vi "enable_channel.vi"(4 "Delay":i32, 6 "V clip":i32, 7 "V att":i32=4095, 8 "error in":errorcluster, 9 "Channel":i32(ring) items=["sendCommand"=9, "FPGA_writeRegister"=3, "FPGA_readRegister"=2, "uC_writeRegister"=1, "uC_readRegister"=0], 10 "id_in":i32, 11 "connection ID":refnum<k5>) -> (0 "error out":errorcluster, 1 "id_out":i32, 3 "connection ID out":refnum<k5>)   [LabVIEW 2009]
doc: "This VI sends a command to the Integration Board and provides the received data when necessary."
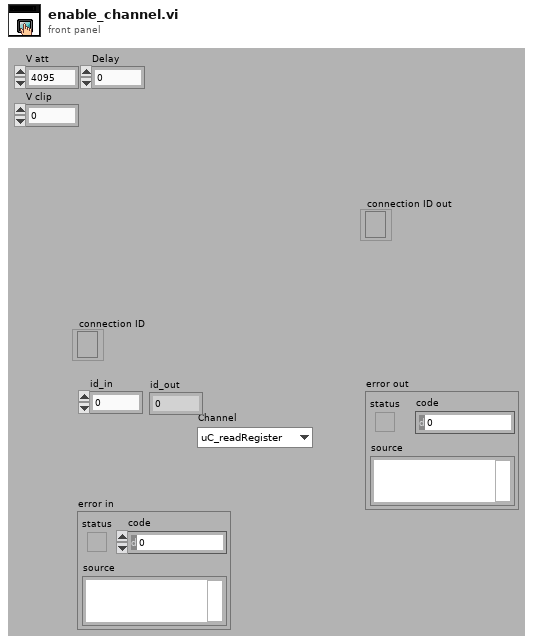
[diagram p1: front panel]
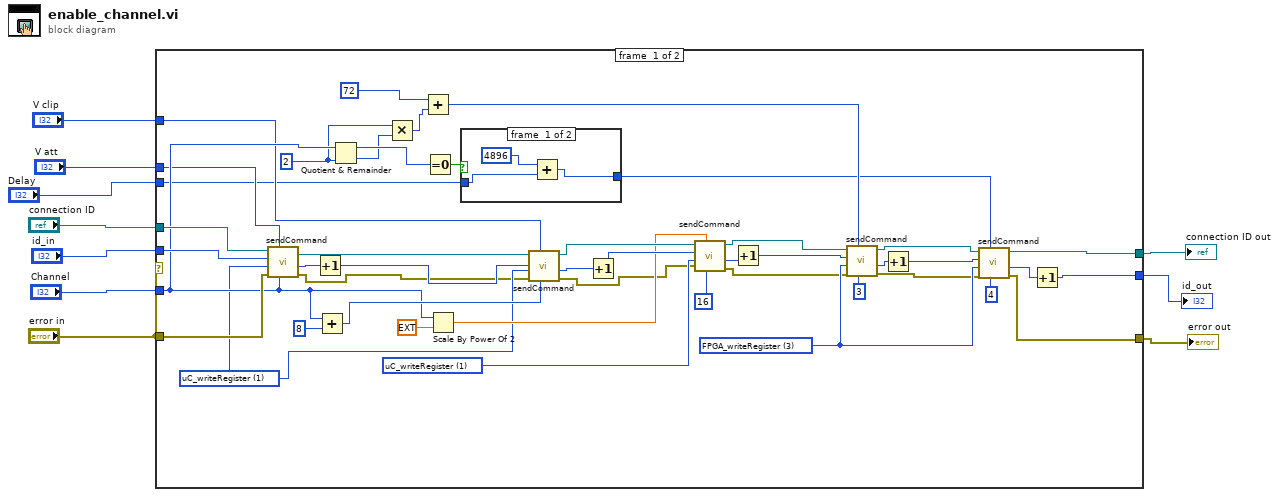
[diagram p0: block diagram]
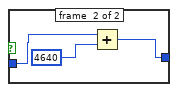
[diagram p2: hidden frame]
diagram:
  n1 = case shown="No Error" "error in" {
    tunnel: "id_in" -> [w53 w62]
    tunnel: "error in" -> [w54 w63]
    tunnel: "connection ID" -> [w55 w64]
    tunnel: [w11 w63] -> w8
    tunnel: [w41 w64] -> w7
    tunnel: "Channel" -> [w28 _]
    tunnel: [w34 w62] -> w4
    tunnel: "V att" -> [w19 _]
    tunnel: "V clip" -> [w18 _]
    tunnel: "Delay" -> [w16 _]
    frame #0 {
      w17 = u16 1 items=["sendCommand"=9, "FPGA_writeRegister"=3, "FPGA_readRegister"=2, "uC_writeRegister"=1, "uC_readRegister"=0] ("Action")
      w20 = u16 1 items=["sendCommand"=9, "FPGA_writeRegister"=3, "FPGA_readRegister"=2, "uC_writeRegister"=1, "uC_readRegister"=0] ("Action")
      w22 = u16 2 ("y")
      w33 = u16 3 items=["sendCommand"=9, "FPGA_writeRegister"=3, "FPGA_readRegister"=2, "uC_writeRegister"=1, "uC_readRegister"=0] ("Action")
      n2 = call "sendCommand.vi"("Address"=w28, "Data"=w19, "error in"=w54, "Action"=w17, "id_in"=w53, "connection ID"=w55) -> ("error out"=w12:errorcluster, "id_out"=w51:i32, "connection ID out"=w48:refnum<k5>)  [unwired: 1 in, 2 out]
      n3 = Increment(x=w51) -> (x+1=w21:i32)
      n4 = Add(x=w28, y=u16 8) -> (x+y=w45:i32)
      n5 = Quotient & Remainder(x=w28, y=w22) -> (x-y*floor(x/y)=w25:i32, floor(x/y)=w24:i32)
      n6 = Multiply(x=w22, y=w24) -> (x*y=w23:i32)
      n7 = Add(x=72 ("Data"), y=w23) -> (x+y=w29:i32)
      n8 = Equal To 0?(x=w25) -> (x = 0?=w27:bool)
      n9 = Scale By Power Of 2(n=w28, x=ext 1.0) -> (x*2^n=w43:ext)
      n10 = case shown="True" w27 {
        tunnel: [w57 w59] -> w26
        tunnel: w16 -> [w56 w60]
        frame #0 {
          n11 = Add(x=4896 ("Data"), y=w56) -> (x+y=w57:i32)
        }
        frame #1 {
          n12 = Add(x=w60, y=4640 ("Data")) -> (x+y=w59:i32)
        }
      }
      n13 = call "sendCommand.vi"("Address"=w45, "Data"=w18, "error in"=w12, "Action"=w17, "id_in"=w21, "connection ID"=w48) -> ("error out"=w13:errorcluster, "id_out"=w52:i32, "connection ID out"=w47:refnum<k5>)  [unwired: 1 in, 2 out]
      n14 = Increment(x=w52) -> (x+1=w50:i32)
      n15 = call "sendCommand.vi"("Address"=16, "Data"=w43, "error in"=w13, "Action"=w20, "id_in"=w50, "connection ID"=w47) -> ("error out"=w14:errorcluster, "id_out"=w49:i32, "connection ID out"=w39:refnum<k5>)  [unwired: 1 in, 2 out]
      n16 = Increment(x=w49) -> (x+1=w38:i32)
      n17 = call "sendCommand.vi"("Address"=3, "Data"=w29, "error in"=w14, "Action"=w33, "id_in"=w38, "connection ID"=w39) -> ("error out"=w15:errorcluster, "id_out"=w36:i32, "connection ID out"=w40:refnum<k5>)  [unwired: 1 in, 2 out]
      n18 = Increment(x=w36) -> (x+1=w37:i32)
      n19 = call "sendCommand.vi"("Address"=4, "Data"=w26, "error in"=w15, "Action"=w33, "id_in"=w37, "connection ID"=w40) -> ("error out"=w11:errorcluster, "id_out"=w35:i32, "connection ID out"=w41:refnum<k5>)  [unwired: 1 in, 2 out]
      n20 = Increment(x=w35) -> (x+1=w34:i32)
    }
    frame #1 {
    }
  }
  "error out" <- w8
  "connection ID out" <- w7
  "id_out" <- w4
